vi "CreateLineOverlay.vi"(7 "error in (no error)":errorcluster, 9 "Bounding rectangle":i32[](array[numeric])) -> (0 "error out":errorcluster, 2 "Lines":T1)   [LabVIEW 2014]
panel:
  # "Right"
  # "Left"
  # "Top"
  # "Bottom"
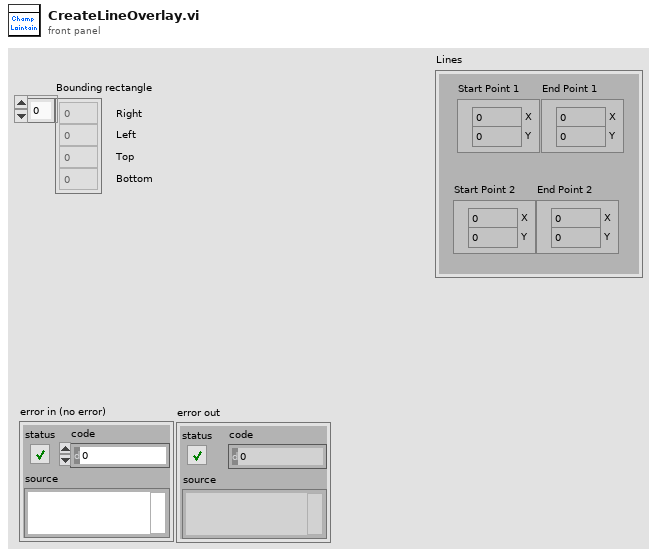
[diagram p1: front panel]
types:
  T1 = cluster{"Start Point 1":cluster{"X":i32, "Y":i32}, "End Point 1":cluster{"X":i32, "Y":i32}, "Start Point 2":cluster{"X":i32, "Y":i32}, "End Point 2":cluster{"X":i32, "Y":i32}}
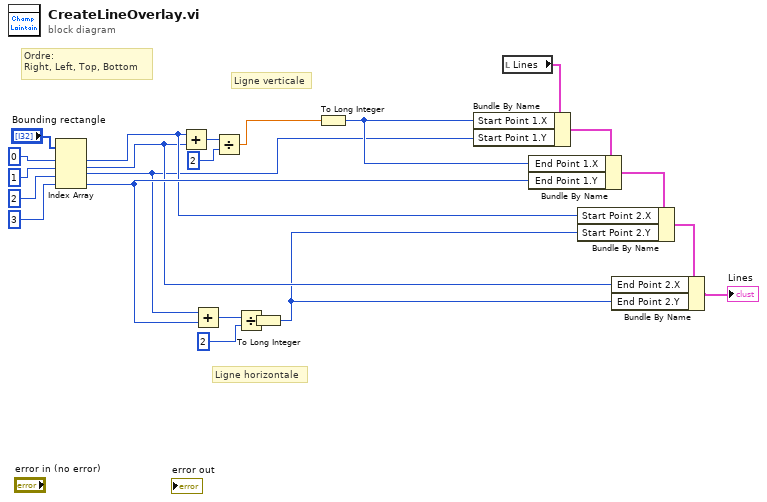
[diagram p0: block diagram]
diagram:
  # "Ligne horizontale"
  # "Ligne verticale"
  # "Ordre:\nRight, Left, Top, Bottom"
  n1 = Index Array(array="Bounding rectangle", index #1=0, index #2=1, index #3=2, index #4=3) -> (element #1=w16:i32, element #2=w14:i32, element #3=w1:i32, element #4=w17:i32)
  n2 = Add(x=w16, y=w14) -> (x+y=w3:i32)
  n3 = Add(x=w1, y=w17) -> (x+y=w8:i32)
  n4 = Divide(x=w3, y=2) -> (x/y=w2:dbl)
  n5 = Divide(x=w8, y=2) -> (x/y=w9:dbl)
  n6 = To Long Integer(number=w9) -> (32bit integer=w5:i32)
  n7 = To Long Integer(number=w2) -> (32bit integer=w6:i32)
  n8 = local read "Lines"() -> (w15:T1)
  n9 = Bundle By Name(cluster=w15, "Start Point 1.X"=w6, "Start Point 1.Y"=w1) -> (w13:T1)
  n10 = Bundle By Name(cluster=w13, "End Point 1.X"=w6, "End Point 1.Y"=w17) -> (w12:T1)
  n11 = Bundle By Name(cluster=w12, "Start Point 2.X"=w16, "Start Point 2.Y"=w5) -> (w11:T1)
  n12 = Bundle By Name(cluster=w11, "End Point 2.X"=w14, "End Point 2.Y"=w5) -> (→"Lines":T1)
